vi "Periodic Tasks.vi"(9 "error in":errorcluster) -> ()   [LabVIEW 2014]
doc: "This VI runs in parallel to other tasks. It can contain as many user-defined periodic loops as you need. These can carry out PID or other sorts of timed response."
uses:
  <vilib>/Rock Robotics/WPI/CAN/TalonSRX/WPI_CANTalonSRX_GlobalStatus.ctl
  <vilib>/Rock Robotics/WPI/Compressor/WPI_CompressorGetSetRefNum.vi
  Drive Global.vi
  Botones Global.vi
  <vilib>/Rock Robotics/WPI/Solenoid/WPI_SolenoidSetEnum.vi
  Robot Global Data.vi
  botones driver.vi
  2283_LED controllers.vi
  <vilib>/Utility/error.llb/Error Cluster From Error Code.vi
  <vilib>/rvi/errors/niLvFpgaAdjustHostInterfaceError.vi
  <vilib>/rvi/interface/nirviReadWriteControl/nirviReadWriteControl.xnode
  <vilib>/Rock Robotics/SystemInterfaces/System/FPGA_SystemFRC FPGA Ref.ctl
  <vilib>/Rock Robotics/SystemInterfaces/roboRIO_FPGA_2015_1.0.10.lvbitx
  Mapa Global.vi
  NiFpgaLv.dll
panel:
  out "Talon Status":T2
  out "current (A)":dbl
  out "Compressor Running":bool
  out "Enabled":bool
  in  "Talon Status":T2
  in  "Elevador":T3
  out "Distance":dbl
  out "Direction":bool
  in  "Axes[0]":dbl
  in  "y":dbl=0.2 format="%#_13g"
  out "LEDs.Radio":u8
  out "LEDs.Comm":u8
  out "LEDs.Mode":u8
  out "LEDs.RSL":bool
  in  "input cluster":T4
  in  "Color":bool
  out "Mapa":cluster{dbl[], dbl[]}(graph)
  in  "X":dbl=350.0
  in  "# de Lecturas":i32=20
  in  "Color":u32(colorbox)
  out "Angular Rate":dbl
  out "Angle":dbl
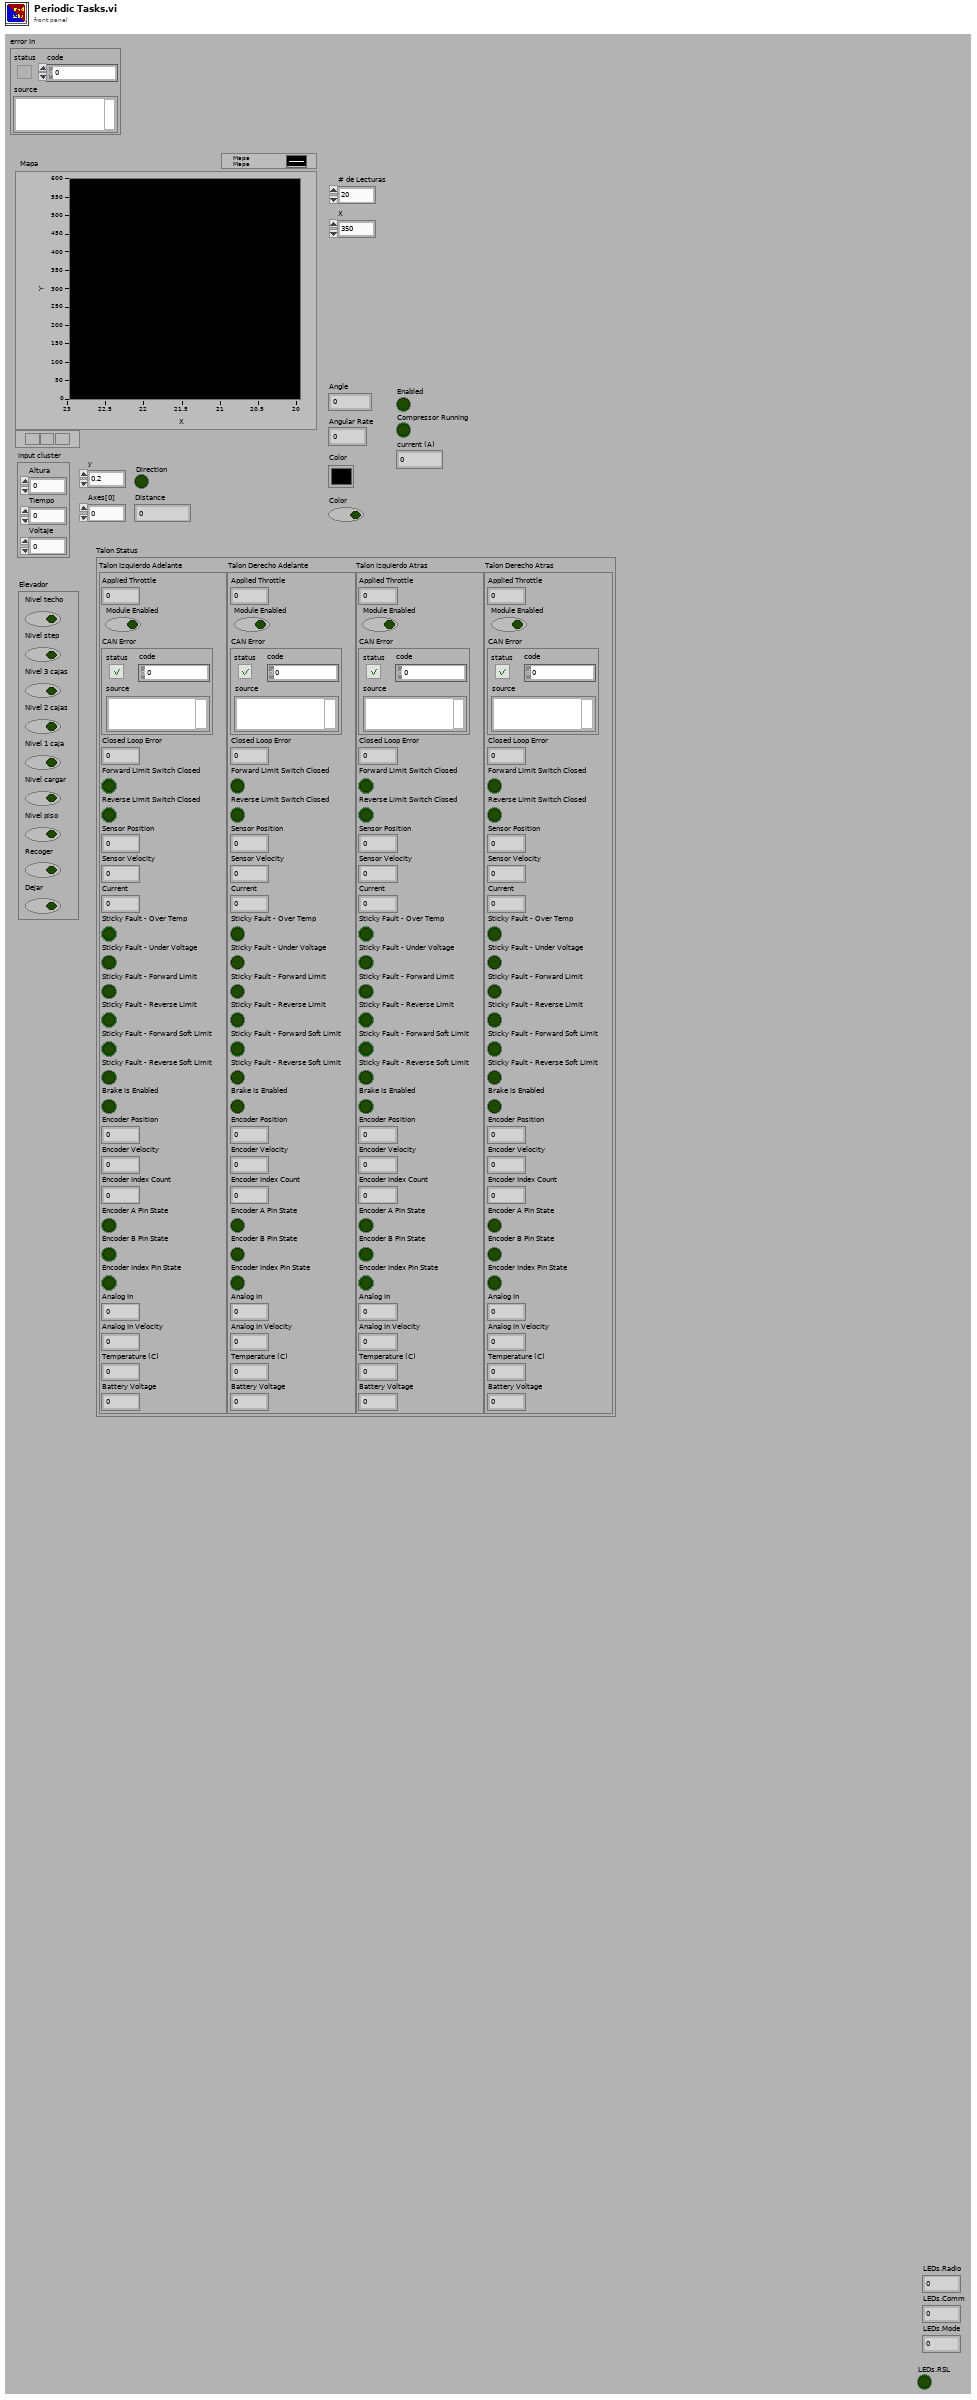
[diagram p1: front panel]
types:
  T1 = typedef "WPI_CANTalonSRX_GlobalStatus.ctl" = cluster{"Applied Throttle":dbl, "Module Enabled":bool, "CAN Error":errorcluster, "Closed Loop Error":dbl, "Forward Limit Switch Closed":bool, "Reverse Limit Switch Closed":bool, "Sensor Position":dbl, "Sensor Velocity":dbl, "Current":dbl, "Sticky Fault - Over Temp":bool, "Sticky Fault - Under Voltage":bool, "Sticky Fault - Forward Limit":bool, "Sticky Fault - Reverse Limit":bool, "Sticky Fault - Forward Soft Limit":bool, "Sticky Fault - Reverse Soft Limit":bool, "Brake is Enabled":bool, "Encoder Position":dbl, "Encoder Velocity":dbl, "Encoder Index Count":dbl, "Encoder A Pin State":bool, "Encoder B Pin State":bool, "Encoder Index Pin State":bool, "Analog In":dbl, "Analog In Velocity":dbl, "Temperature (C)":dbl, "Battery Voltage":dbl}
  T2 = cluster{"Talon Izquierdo Adelante":T1, "Talon Derecho Adelante":T1, "Talon Izquierdo Atras":T1, "Talon Derecho Atras":T1}
  T3 = cluster{"Nivel techo":bool, "Nivel step":bool, "Nivel 3 cajas":bool, "Nivel 2 cajas":bool, "Nivel 1 caja":bool, "Nivel cargar":bool, "Nivel piso":bool, "Recoger":bool, "Dejar":bool}
  T4 = cluster{"Altura":dbl, "Tiempo":dbl, "Voltaje":dbl}
  T5 = typedef "WPI_I2CDevRef.ctl" = cluster{"DevStatus":errorcluster, "Controller":T6, "Device Address":u8, "Handle":i32, "I2C Bus":T7}
  T6 = typedef "FPGA_TypedefDigitalModule.ctl" = enum16{"Controller 1"}
  T7 = typedef "i2c_bus.ctl" = enum16{"I2C On-Board", "I2C MXP", "Invalid"}
  T8 = cluster{"botones":cluster{"Buttons[0]":bool, "Buttons[1]":bool, "Buttons[2]":bool, "Buttons[3]":bool, "Buttons[4]":bool, "Buttons[5]":bool, "Buttons[6]":bool, "Buttons[7]":bool, "Buttons[8]":bool}, "cluster":cluster{"Axes[0]":dbl, "Axes[1]":dbl, "Axes[2]":dbl, "Axes[3]":dbl, "Axes[4]":dbl, "Axes[5]":dbl, "Axes[6]":dbl, "Axes[7]":dbl, "Axes[8]":dbl}}
  T9 = typedef "WPI_DriverStationRobotMode2.ctl" = enum16{"Autonomous Disabled", "Autonomous Enabled", "Teleop Disabled", "Teleop Enabled", "Disconnected", "Finish", "Test Disabled", "Test Enabled", "Emergency Stopped"}
  T10 = typedef "WPI_GyroDevRef.ctl" = cluster{"DevStatus":errorcluster, "Analog Module":T11, "Analog Channel":T12, "Offset":dbl, "Gain (VoltsPerDegree/Second)":dbl}
  T11 = typedef "FPGA_TypedefAnalogModule.ctl" = enum16{"Controller 1"}
  T12 = typedef "FPGA_AIChannel.ctl" = enum8{"AI 0", "AI 1", "AI 2", "AI 3", "AI MXP 0", "AI MXP 1", "AI MXP 2", "AI MXP 3", "Invalid"}
  T13 = typedef "WPI_CompressorDevRef.ctl" = cluster{"DevStatus":errorcluster, "Pneumatics Control Module":u8}
  T14 = typedef "WPI_AccelerometerDevRef.ctl" = cluster{"DevStatus":errorcluster, "Controller":T11, "Scaling":T15, "Analog Channels":T16, "I2C Bus":T7, "SPI Bus":T17, "Accel Range":T18, "ADXL345 Axes":T19, "Handle":i32, "Device Address":u8, "Accel Type":enum16{"Analog", "ADXL345 I2C", "ADXL345 SPI", "Internal"}}
  T15 = typedef "WPI_AccelerometerScaling.ctl" = cluster{"Gain (VoltsPerG)":dbl, "Center Voltage":dbl}
  T16 = typedef "WPI_AccelerometerAnalogChannels.ctl" = cluster{"X-Axis":T12, "Y-Axis":T12, "Z-Axis":T12}
  T17 = typedef "spi_bus.ctl" = enum16{"SPI On-Board, CS0", "SPI On-Board, CS1", "SPI On-Board, CS2", "SPI On-Board, CS3", "SPI MXP", "Invalid"}
  T18 = typedef "ADXL345 Range.ctl" = u8
  T19 = typedef "WPI_AccelerometerADXL345 Axes.ctl" = cluster{"X-Axis":bool, "Y-Axis":bool, "Z-Axis":bool}
  T20 = cluster{"Buttons[0]":bool, "Buttons[1]":bool, "Buttons[2]":bool, "Buttons[3]":bool, "Buttons[4]":bool, "Buttons[5]":bool, "Buttons[6]":bool, "Buttons[7]":bool, "Buttons[8]":bool}
  T21 = cluster{"Axes[0]":dbl, "Axes[1]":dbl, "Axes[2]":dbl, "Axes[3]":dbl, "Axes[4]":dbl, "Axes[5]":dbl, "Axes[6]":dbl, "Axes[7]":dbl, "Axes[8]":dbl}
  T22 = cluster{"X-Axis":dbl, "Y-Axis":dbl, "Z-Axis":dbl}
  T23 = typedef "WPI_EncoderDevRef.ctl" = cluster{"DevStatus":errorcluster, "EncoderIndex":T24, "CounterIndex":T25, "DistancePerCount":dbl, "Decoding Type":T26}
  T24 = typedef "FPGA_EncoderIdx.ctl" = enum8{"Enc 0", "Enc 1", "Enc 2", "Enc 3", "Enc 4", "Enc 5", "Enc 6", "Enc 7", "Invalid"}
  T25 = typedef "FPGA_CounterCtrSystemIndex.ctl" = enum8{"Ctr 0", "Ctr 1", "Ctr 2", "Ctr 3", "Ctr 4", "Ctr 5", "Ctr 6", "Ctr 7", "Invalid"}
  T26 = typedef "WPI_EncoderType.ctl" = enum16{"1x", "2x", "4x"}
  T27 = typedef "WPI_MotorControlDeviceRef.ctl" = cluster{"DeviceStatus":errorcluster, "Type":T28, "PWM":cluster{"Controller":T6, "PWM Channel":T29, "DeadBand":T30}, "CAN":cluster{"Device Number":u8, "Control Mode":T31, "Semaphore":T32, "Max Vout":dbl, "TalonSRX Control Mode":T33}, "Invert":bool, "TransformRef":T34, "InvTransformRef":T34}
  T28 = typedef "WPI_MotorControlType.ctl" = enum16{"PWM", "CAN", "CANTalonSRX"}
  T29 = typedef "FPGA_DIOPWMChannel.ctl" = enum8{"PWM 0", "PWM 1", "PWM 2", "PWM 3", "PWM 4", "PWM 5", "PWM 6", "PWM 7", "PWM 8", "PWM 9", "PWM MXP 0", "PWM MXP 1", "PWM MXP 2", "PWM MXP 3", "PWM MXP 4", "PWM MXP 5", "PWM MXP 6", "PWM MXP 7", "PWM MXP 8", "PWM MXP 9", "Invalid"}
  T30 = typedef "WPI_PWMDeadband.ctl" = cluster{"Name":string, "maxPositivePwm":i32, "minPositivePwm":i32, "centerPwm":i32, "maxNegativePwm":i32, "minNegativePwm":i32, "angularRange":u16}
  T31 = typedef "WPI_CANJaguar_ControlMode.ctl" = enum8{"Percent VBus", "Current", "Speed", "Position", "Voltage"}
  T32 = typedef "Semaphore RefNum" = refnum<k1>
  T33 = typedef "WPI_CANTalonSRX_APIControlMode.ctl" = enum8{"Percent VBus", "Speed", "Position", "Slave", "Unchanged / Invalid"}
  T34 = typedef "WPI_PWMTransform_ConPane.ctl" = refnum<vi>
  T35 = typedef "WPI_SolenoidValue.ctl" = enum16{"Off", "On", "Forward", "Reverse"}
  T36 = typedef "WPI_SolenoidDevRef.ctl" = cluster{"DevStatus":errorcluster, "Pneumatics Control Module":u8, "Forward Solenoid Channel":T37, "Reverse Solenoid Channel":T37}
  T37 = typedef "WPI_SolenoidChannel.ctl" = enum8{"Solenoid 0", "Solenoid 1", "Solenoid 2", "Solenoid 3", "Solenoid 4", "Solenoid 5", "Solenoid 6", "Solenoid 7", "Invalid"}
  T38 = typedef "FPGA_SystemFRC FPGA Ref.ctl" = refnum<k20>
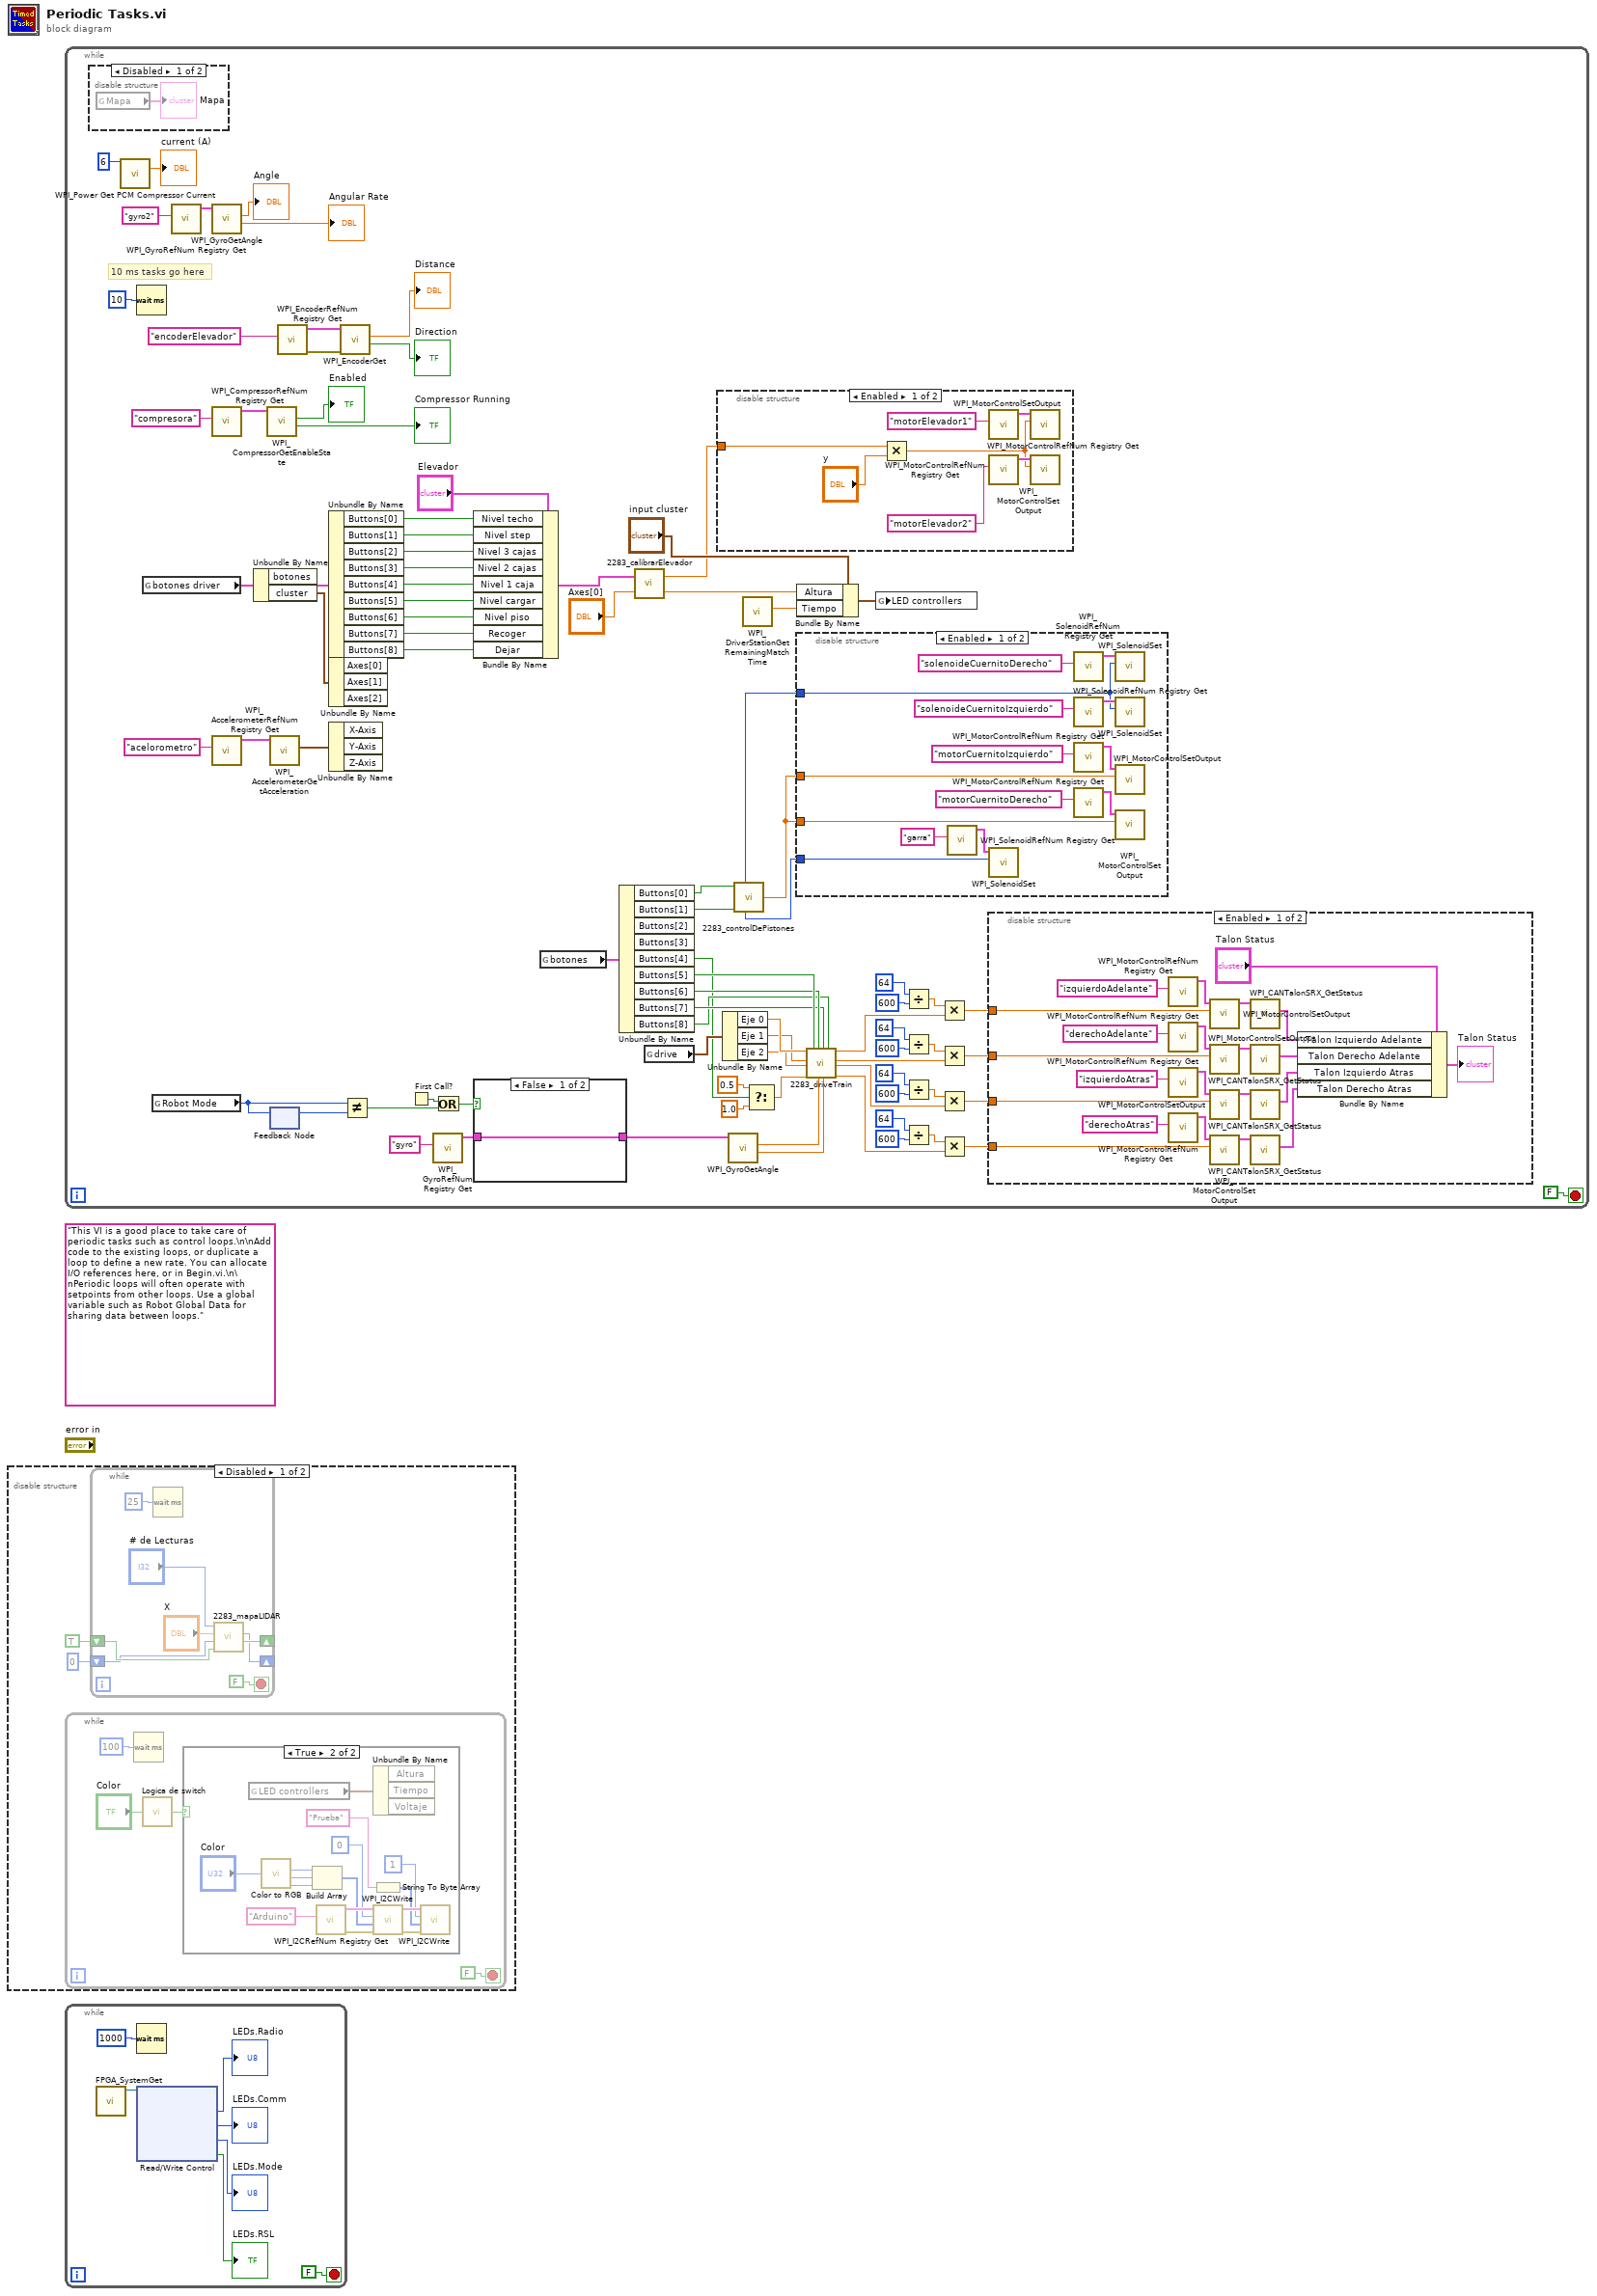
[diagram p0: block diagram]
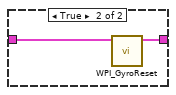
[diagram p8: hidden frame]
diagram:
  (unwired) "This VI is a good place to take care of periodic tasks such as control loops.\n\nAdd code to the existing loops, or duplicate a loop to define a new rate. You can allocate I/O references here, or in Begin.vi.\n\nPeriodic loops will often operate with setpoints from other loops. Use a global variable such as Robot Global Data for sharing data between loops."
  n1 = disable-structure shown="Disabled" {
    frame Disabled {
      n2 = while {
        stop <- FALSE stop-if-true
        n3 = Wait (ms)(milliseconds to wait=u32 100 ("millisecond timer value")) -> ()  [unwired: 1 out]
        n4 = call "Logica de switch.vi"("Input"="Color") -> ("Output"=w3:bool)
        n5 = case shown="True" w3 {
          frame False {
          }
          frame True {
            n6 = global read "2283_LED controllers.vi" "LED controllers"() -> (w7:T4)
            n7 = call <vilib>:"Color to RGB.vi"("Color"="Color") -> ("R"=w15:u8, "G"=w14:u8, "B"=w13:u8)  [unwired: 1 out]
            n8 = Build Array(w15, w14, w13) -> (w16:u8[])
            n9 = call <vilib>:"WPI_I2CRefNum Registry Get.vi"("refnum name"="Arduino") -> ("error out"=w18:errorcluster, "I2CDevRef"=w19:T5)  [unwired: 9 in]
            n10 = Unbundle By Name(w7) -> ()  [unwired: 3 out]
            n11 = String To Byte Array(string="Prueba") -> (unsigned byte array=w9:u8[])
            n12 = call <vilib>:"WPI_I2CWrite.vi"("error in (no error)"=w18, "I2CDataToSend"=w16, "I2CRegister"=u8 0 ("Data To Send"), "I2CDevRef"=w19) -> ("error out"=w11:errorcluster, "I2CDevRef"=w12:T5)  [unwired: 6 in]
            n13 = call <vilib>:"WPI_I2CWrite.vi"("error in (no error)"=w11, "I2CDataToSend"=w9, "I2CRegister"=u8 1 ("Data To Send"), "I2CDevRef"=w12) -> ()  [unwired: 6 in, 2 out]
          }
        }
      }
      n14 = while {
        shift-right: [w24] -> _
        shift-left: 0 -> [w26]
        shift-right: [w25] -> _
        shift-left: TRUE -> [w27]
        stop <- FALSE stop-if-true
        n15 = Wait (ms)(milliseconds to wait=u32 25 ("millisecond timer value")) -> ()  [unwired: 1 out]
        n16 = call "2283_mapaLIDAR.vi"("Boolean Shift Register In"=w27, "Numeric Shift Register In"=w26, "X"="X", "# de Lecturas"="# de Lecturas") -> ("Boolean Shift Register Out"=w25:bool, "Num Shift Register Out"=w24:i32)  [unwired: 4 in]
      }
    }
    frame Enabled {
    }
  }
  n17 = while {
    stop <- FALSE stop-if-true
    # "10 ms tasks go here"
    n18 = disable-structure shown="Disabled" {
      frame Disabled {
        n19 = global read "Mapa Global.vi" "Mapa"() -> (→"Mapa":cluster{dbl[], dbl[]})
      }
      frame Enabled {
      }
    }
    n20 = call <vilib>:"WPI_Power Get PCM Compressor Current.vi"("Pneumatics Control Module (0)"=u8 6) -> ("current (A)"=→"current (A)":dbl)  [unwired: 13 in, 1 out]
    n21 = Wait (ms)(milliseconds to wait=u32 10) -> ()  [unwired: 1 out]
    n22 = global read "botones driver.vi" "botones driver"() -> (w90:T8)
    n23 = global read "Robot Global Data.vi" "Robot Mode"() -> (w97:T9)
    n24 = call <vilib>:"WPI_GyroRefNum Registry Get.vi"("refnum name"="gyro2") -> ("GyroDevRef"=w84:T10)  [unwired: 9 in, 1 out]
    n25 = call <vilib>:"WPI_GyroGetAngle.vi"("GyroDevRef"=w84) -> ("Angular Rate"=→"Angular Rate":dbl, "Angle"=→"Angle":dbl)  [unwired: 7 in, 2 out]
    n26 = call <vilib>:"WPI_CompressorRefNum Registry Get.vi"("refnum name"="compresora") -> ("CompressorDevRef"=w56:T13)  [unwired: 9 in, 1 out]
    n27 = call <vilib>:"WPI_AccelerometerRefNum Registry Get.vi"("refnum name"="acelorometro") -> ("AccelerometerDevRef"=w81:T14)  [unwired: 9 in, 1 out]
    n28 = Unbundle By Name(w90) -> ("botones"=w89:T20, "cluster"=w88:T21)
    n29 = call <vilib>:"WPI_CompressorGetEnableState.vi"("CompressorDevRef"=w56) -> ("Compressor Running"=→"Compressor Running":bool, "Enabled"=→"Enabled":bool)  [unwired: 7 in, 2 out]
    n30 = call <vilib>:"WPI_AccelerometerGetAcceleration.vi"("AccelerometerDevRef"=w81) -> ("Accelerations"=w79:T22)  [unwired: 8 in, 2 out]
    n31 = feedback-in #1(w97) -> ()
    n32 = feedback #1() -> (w98:T9)  [unwired: 1 in]
    n33 = call <vilib>:"WPI_EncoderRefNum Registry Get.vi"("refnum name"="encoderElevador") -> ("error out"=w74:errorcluster, "EncoderDevRef"=w73:T23)  [unwired: 9 in]
    n34 = Unbundle By Name(w89) -> ("Buttons[0]"=w65:bool, "Buttons[1]"=w64:bool, "Buttons[2]"=w63:bool, "Buttons[3]"=w62:bool, "Buttons[4]"=w61:bool, "Buttons[5]"=w60:bool, "Buttons[6]"=w59:bool, "Buttons[7]"=w58:bool, "Buttons[8]"=w30:bool)
    n35 = Unbundle By Name(w88) -> ()  [unwired: 3 out]
    n36 = Unbundle By Name(w79) -> ()  [unwired: 3 out]
    n37 = call <vilib>:"WPI_EncoderGet.vi"("error in (no error)"=w74, "EncoderDevRef"=w73) -> ("Direction"=→"Direction":bool, "Distance"=→"Distance":dbl)  [unwired: 4 in, 4 out]
    n38 = Not Equal?(x=w97, y=w98) -> (x != y?=w96:bool)
    n39 = First Call?() -> (First Call?: T/F=w99:bool)
    n40 = call <vilib>:"WPI_GyroRefNum Registry Get.vi"("refnum name"="gyro") -> ("GyroDevRef"=w102:T10)  [unwired: 9 in, 1 out]
    n41 = Or(x=w99, y=w96) -> (x .or. y?=w100:bool)
    n42 = Bundle By Name(cluster="Elevador", "Nivel techo"=w65, "Nivel step"=w64, "Nivel 3 cajas"=w63, "Nivel 2 cajas"=w62, "Nivel 1 caja"=w61, "Nivel cargar"=w60, "Nivel piso"=w59, "Recoger"=w58, "Dejar"=w30) -> (w67:T3)
    n43 = case shown="False" w100 {
      tunnel: w102 -> [w162 w164]
      tunnel: [w162 w163] -> w101
      frame False {
      }
      frame True {
        n44 = call <vilib>:"WPI_GyroReset.vi"("GyroDevRef"=w164) -> ("GyroDevRef"=w163:T10)  [unwired: 9 in, 1 out]
      }
    }
    n45 = global read "Botones Global.vi" "botones"() -> (w107:T20)
    n46 = Unbundle By Name(w107) -> ("Buttons[0]"=w87:bool, "Buttons[1]"=w86:bool, "Buttons[4]"=w94:bool, "Buttons[5]"=w106:bool, "Buttons[6]"=w105:bool, "Buttons[7]"=w104:bool, "Buttons[8]"=w103:bool)  [unwired: 2 out]
    n47 = call "2283_calibrarElevador.vi"("Potenciometro linear"="Axes[0]", "input cluster"=w67) -> ("Altura"=w66:dbl, "Output elevador"=w70:dbl)
    n48 = global read "Drive Global.vi" "drive"() -> (w115:cluster{"Eje 0":dbl, "Eje 1":dbl, "Eje 2":dbl})
    n49 = disable-structure shown="Enabled" {
      disable-tunnel: w70 -> [w157 _]
      frame Enabled {
        n50 = Multiply(x=w157, y="y") -> (x*y=w156:dbl)
        n51 = call <vilib>:"WPI_MotorControlRefNum Registry Get.vi"("refnum name"="motorElevador1") -> ("MotorControlDevRef"=w158:T27)  [unwired: 9 in, 1 out]
        n52 = call <vilib>:"WPI_MotorControlRefNum Registry Get.vi"("refnum name"="motorElevador2") -> ("MotorControlDevRef"=w160:T27)  [unwired: 9 in, 1 out]
        n53 = call <vilib>:"WPI_MotorControlSetOutput.vi"("Output"=w156, "MotorControlDevRef"=w158) -> ()  [unwired: 7 in, 3 out]
        n54 = call <vilib>:"WPI_MotorControlSetOutput.vi"("Output"=w156, "MotorControlDevRef"=w160) -> ()  [unwired: 7 in, 3 out]
      }
      frame Disabled {
      }
    }
    n55 = Unbundle By Name(w115) -> ("Eje 0"=w112:dbl, "Eje 1"=w111:dbl, "Eje 2"=w110:dbl)
    n56 = call <vilib>:"WPI_GyroGetAngle.vi"("GyroDevRef"=w101) -> ("Angular Rate"=w108:dbl, "Angle"=w109:dbl)  [unwired: 7 in, 2 out]
    n57 = call "2283_controlDePistones.vi"("Boton 1"=w87, "Boton 2"=w86) -> ("solenoideCuernito"=w113:T35, "solenoideGarra"=w114:T35, "Motor"=w57:dbl)  [unwired: 4 in]
    n58 = call <vilib>:"WPI_DriverStationGetRemainingMatchTime.vi"() -> ("Match Time(s)"=w76:sgl)  [unwired: 10 in, 1 out]
    n59 = Select(t=0.5, s=w94, f=1.0 ("Potenciometro")) -> (s? t:f=w92:dbl)
    n60 = Bundle By Name(cluster="input cluster", "Altura"=w66, "Tiempo"=w76) -> (w77:T4)
    n61 = disable-structure shown="Enabled" {
      disable-tunnel: w57 -> [w142 _]
      disable-tunnel: w114 -> [w144 _]
      disable-tunnel: w113 -> [w143 _]
      disable-tunnel: w57 -> [w141 _]
      frame Enabled {
        n62 = call <vilib>:"WPI_SolenoidRefNum Registry Get.vi"("refnum name"="garra") -> ("SolenoidDevRef"=w146:T36)  [unwired: 9 in, 1 out]
        n63 = call-poly <vilib>:"WPI_SolenoidSet.vi"("Value"=w144, "SolenoidDevRef"=w146) -> ()  [unwired: 8 in, 2 out]
        n64 = call <vilib>:"WPI_SolenoidRefNum Registry Get.vi"("refnum name"="solenoideCuernitoDerecho") -> ("SolenoidDevRef"=w147:T36)  [unwired: 9 in, 1 out]
        n65 = call <vilib>:"WPI_SolenoidRefNum Registry Get.vi"("refnum name"="solenoideCuernitoIzquierdo") -> ("SolenoidDevRef"=w149:T36)  [unwired: 9 in, 1 out]
        n66 = call <vilib>:"WPI_MotorControlRefNum Registry Get.vi"("refnum name"="motorCuernitoIzquierdo") -> ("MotorControlDevRef"=w152:T27)  [unwired: 9 in, 1 out]
        n67 = call <vilib>:"WPI_MotorControlRefNum Registry Get.vi"("refnum name"="motorCuernitoDerecho") -> ("MotorControlDevRef"=w151:T27)  [unwired: 9 in, 1 out]
        n68 = call-poly <vilib>:"WPI_SolenoidSet.vi"("Value"=w143, "SolenoidDevRef"=w147) -> ()  [unwired: 8 in, 2 out]
        n69 = call-poly <vilib>:"WPI_SolenoidSet.vi"("Value"=w143, "SolenoidDevRef"=w149) -> ()  [unwired: 8 in, 2 out]
        n70 = call <vilib>:"WPI_MotorControlSetOutput.vi"("Output"=w142, "MotorControlDevRef"=w152) -> ()  [unwired: 7 in, 3 out]
        n71 = call <vilib>:"WPI_MotorControlSetOutput.vi"("Output"=w141, "MotorControlDevRef"=w151) -> ()  [unwired: 7 in, 3 out]
      }
      frame Disabled {
      }
    }
    n72 = call "2283_driveTrain.vi"("y"=w112, "x"=w111, "g"=w110, "p"=w92, "Boton 1"=w106, "Boton 2"=w105, "angulo"=w109, "Boton 3"=w104, "angle rate"=w108, "Modificador"=w103) -> ("i1"=w47:dbl, "d1"=w42:dbl, "i2"=w37:dbl, "d2"=w32:dbl)  [unwired: 6 in]
    n73 = global write "2283_LED controllers.vi" "LED controllers"(w77) -> ()
    n74 = Divide(x=64, y=600) -> (x/y=w48:dbl)
    n75 = Divide(x=64, y=600) -> (x/y=w43:dbl)
    n76 = Divide(x=64, y=600) -> (x/y=w38:dbl)
    n77 = Divide(x=64, y=600) -> (x/y=w33:dbl)
    n78 = Multiply(x=w48, y=w47) -> (x*y=w46:dbl)
    n79 = Multiply(x=w43, y=w42) -> (x*y=w41:dbl)
    n80 = Multiply(x=w38, y=w37) -> (x*y=w36:dbl)
    n81 = Multiply(x=w33, y=w32) -> (x*y=w31:dbl)
    n82 = disable-structure shown="Enabled" {
      disable-tunnel: w46 -> [w119 _]
      disable-tunnel: w41 -> [w120 _]
      disable-tunnel: w36 -> [w121 _]
      disable-tunnel: w31 -> [w122 _]
      frame Enabled {
        n83 = call <vilib>:"WPI_MotorControlRefNum Registry Get.vi"("refnum name"="izquierdoAdelante") -> ("MotorControlDevRef"=w140:T27)  [unwired: 9 in, 1 out]
        n84 = call <vilib>:"WPI_MotorControlRefNum Registry Get.vi"("refnum name"="derechoAdelante") -> ("MotorControlDevRef"=w136:T27)  [unwired: 9 in, 1 out]
        n85 = call <vilib>:"WPI_MotorControlRefNum Registry Get.vi"("refnum name"="izquierdoAtras") -> ("MotorControlDevRef"=w129:T27)  [unwired: 9 in, 1 out]
        n86 = call <vilib>:"WPI_MotorControlRefNum Registry Get.vi"("refnum name"="derechoAtras") -> ("MotorControlDevRef"=w138:T27)  [unwired: 9 in, 1 out]
        n87 = call <vilib>:"WPI_MotorControlSetOutput.vi"("Output"=w119, "MotorControlDevRef"=w140) -> ("MotorControlDevRef"=w134:T27)  [unwired: 7 in, 2 out]
        n88 = call <vilib>:"WPI_MotorControlSetOutput.vi"("Output"=w120, "MotorControlDevRef"=w136) -> ("MotorControlDevRef"=w133:T27)  [unwired: 7 in, 2 out]
        n89 = call <vilib>:"WPI_MotorControlSetOutput.vi"("Output"=w121, "MotorControlDevRef"=w129) -> ("MotorControlDevRef"=w131:T27)  [unwired: 7 in, 2 out]
        n90 = call <vilib>:"WPI_MotorControlSetOutput.vi"("Output"=w122, "MotorControlDevRef"=w138) -> ("MotorControlDevRef"=w132:T27)  [unwired: 7 in, 2 out]
        n91 = call <vilib>:"WPI_CANTalonSRX_GetStatus.vi"("CAN Talon SRX Ref"=w134) -> ("Talon SRX Status"=w127:T1)  [unwired: 8 in, 2 out]
        n92 = call <vilib>:"WPI_CANTalonSRX_GetStatus.vi"("CAN Talon SRX Ref"=w133) -> ("Talon SRX Status"=w126:T1)  [unwired: 8 in, 2 out]
        n93 = call <vilib>:"WPI_CANTalonSRX_GetStatus.vi"("CAN Talon SRX Ref"=w131) -> ("Talon SRX Status"=w125:T1)  [unwired: 8 in, 2 out]
        n94 = call <vilib>:"WPI_CANTalonSRX_GetStatus.vi"("CAN Talon SRX Ref"=w132) -> ("Talon SRX Status"=w124:T1)  [unwired: 8 in, 2 out]
        n95 = Bundle By Name(cluster="Talon Status", "Talon Izquierdo Adelante"=w127, "Talon Derecho Adelante"=w126, "Talon Izquierdo Atras"=w125, "Talon Derecho Atras"=w124) -> (→"Talon Status":T2)
      }
      frame Disabled {
      }
    }
  }
  n96 = while {
    stop <- FALSE stop-if-true
    n97 = call <vilib>:"FPGA_SystemGet.vi"() -> ("FRC FPGA Ref"=w171:T38)  [unwired: 11 in]
    n98 = Wait (ms)(milliseconds to wait=u32 1000) -> ()  [unwired: 1 out]
    n99 = xnode "Read/Write Control"("FPGA VI Reference In"=w171) -> ("LEDs.Radio"=→"LEDs.Radio":u8, "LEDs.Comm"=→"LEDs.Comm":u8, "LEDs.Mode"=→"LEDs.Mode":u8, "LEDs.RSL"=→"LEDs.RSL":bool)  [unwired: 1 in, 2 out]
  }
